vi "log_debug.vi"(8 "error in (no error)":errorcluster, 11 "message":string) -> (0 "error out":errorcluster)   [LabVIEW 2021, in "system.logging.lvclass"]
uses:
  system.logging.lvclass
  system.logging.lvclass/system.logging.ctl
  severity.ctl
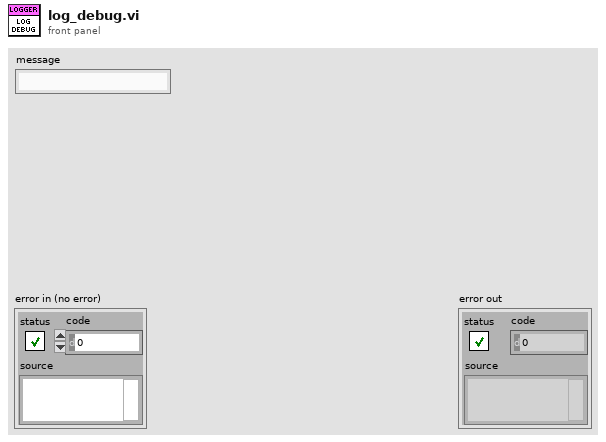
[diagram p1: front panel]
types:
  T1 = typedef "system.logging.lvclass/severity.ctl" = enum8{"trace", "debug", "info", "warning", "error"}
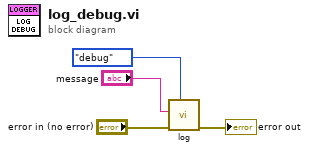
[diagram p0: block diagram]
diagram:
  n1 = call "log.vi"("severity"=severity."debug", "error in (no error)"="error in (no error)", "message"="message") -> ("error out"=→"error out":errorcluster)  [unwired: 8 in]
